vi "InitObjects.vi"(0 "Stand":refnum<class "Stand.lvclass">, 11 "error in":errorcluster, 13 "FPGA API":refnum<class "FPGA API.lvclass">) -> (4 "Stand out":refnum<class "Stand.lvclass">, 15 "error out":errorcluster)   [LabVIEW 2019, in "Stand.lvclass"]
uses:
  Stand.lvclass
  C:/Users/H4001/Documents/GitHub/H4000/src/Proccess_class/Proccess.lvclass
  C:/Users/H4001/Documents/GitHub/H4000/src/Device_class/Device.lvclass
  FPGA_API_class/FPGA API.lvclass
  Device_class/Device.lvclass/Device.ctl
  Proccess_class/Proccess.lvclass/Proccess.ctl
  AI_class/AI.lvclass
  Stand.lvclass/Stand.ctl
  Sig_DI_Simple_class/Sig_DI_Simple.lvclass
  MessageAMC_class/MessageAMC.lvclass
  C:/Users/H4001/Documents/GitHub/H4000/src/MessageInterface_class/MessageInterface.lvclass
  PM_Group_class/PM_Group.lvclass
  FPGA/TypeDef/DO index.ctl
  FPGA/TypeDef/DI index.ctl
  Valve_2DO_2DI_class/Valve_2DO_2DI.lvclass
  Proccess_class/Proccess.lvclass
  NeedleValve_class/NeedleValve.lvclass
  Device_class/Device.lvclass
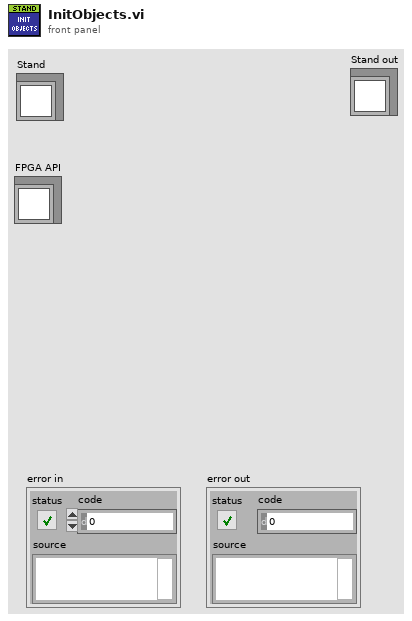
[diagram p1: front panel]
types:
  T1 = enum16{"AI", "DI", "NV", "PM", "VLV 44.1 44.2"}[]
  T2 = typedef "DI index.ctl" = u8
  T3 = typedef "DO index.ctl" = u8
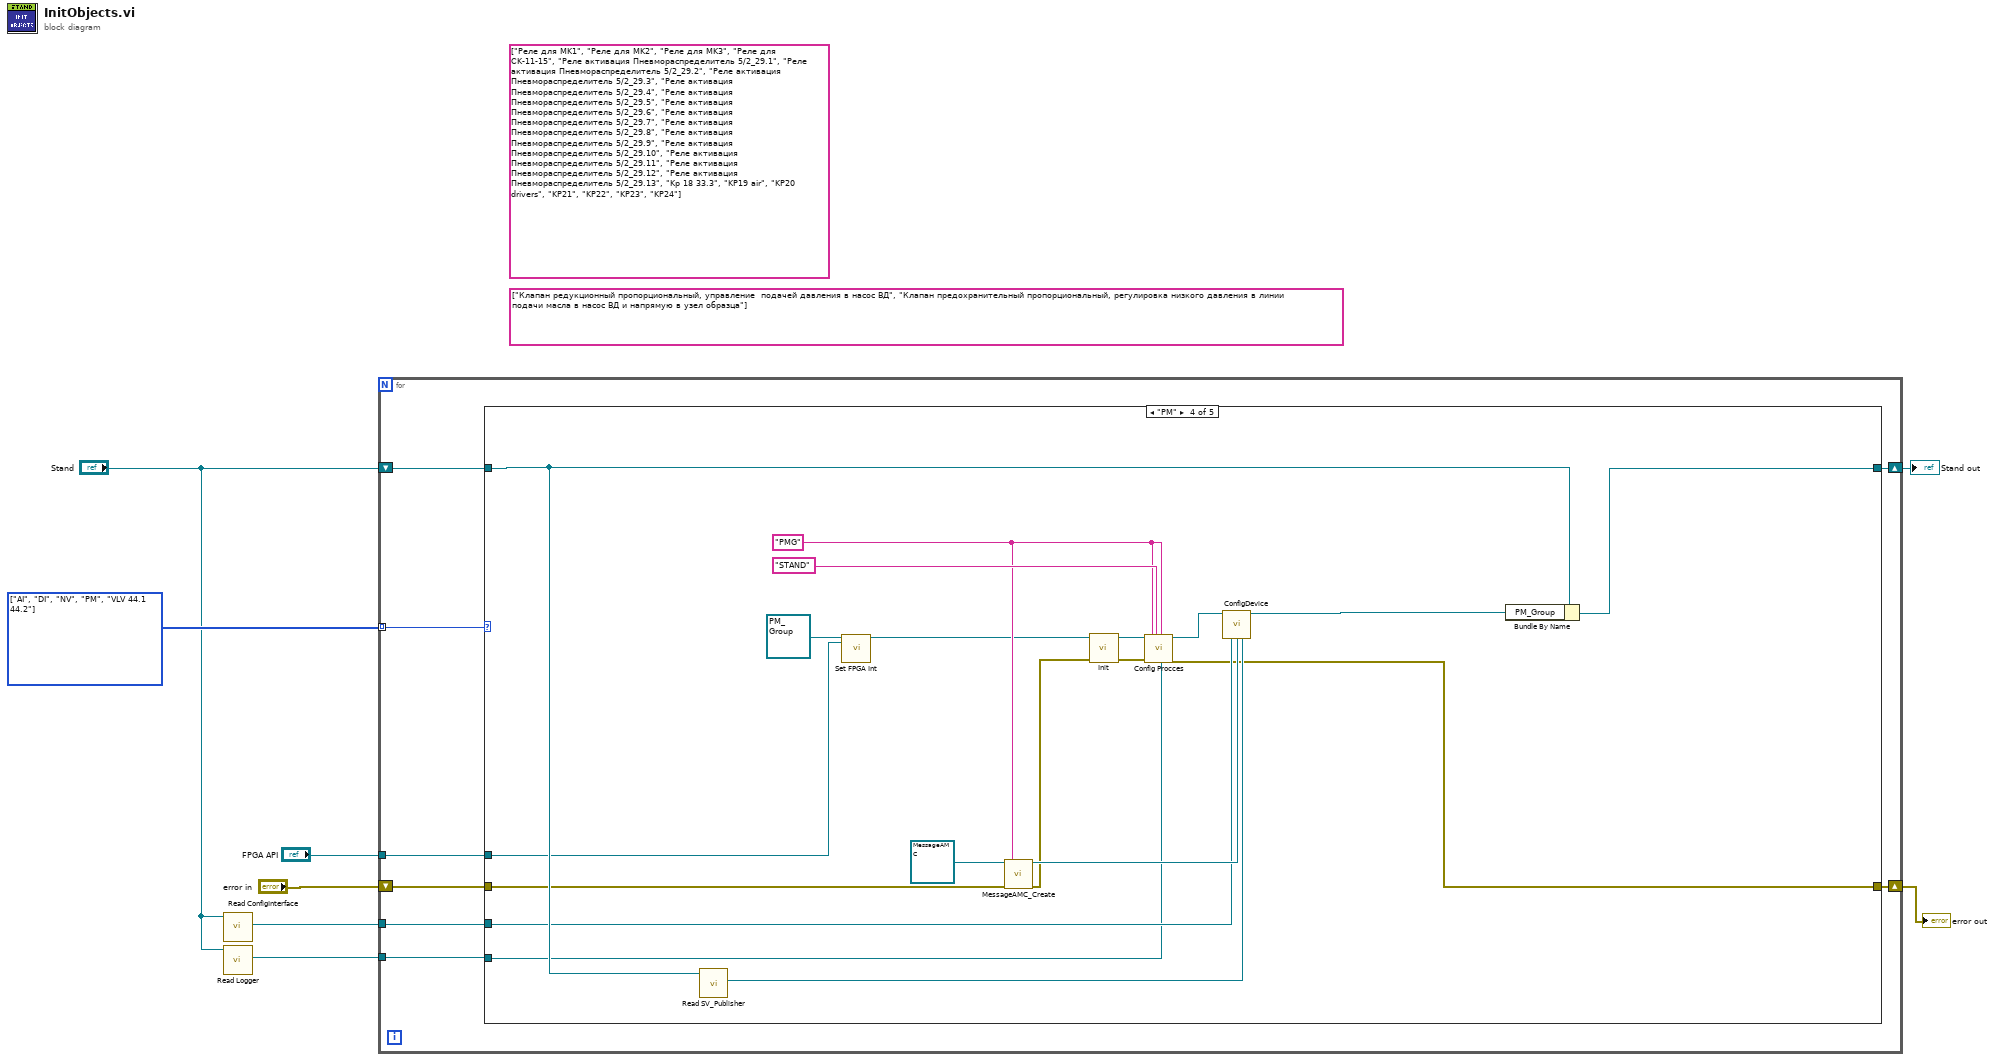
[diagram p0: block diagram]
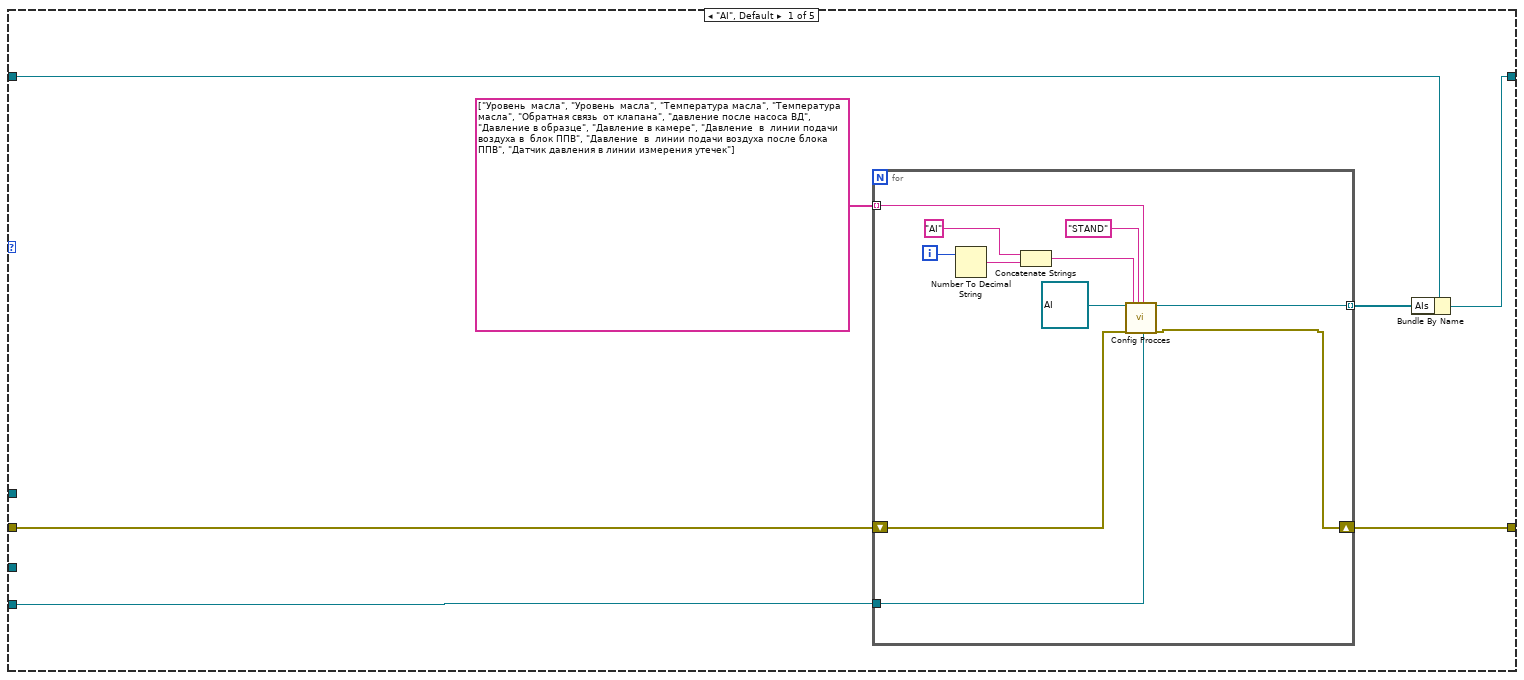
[diagram p2: hidden frame]
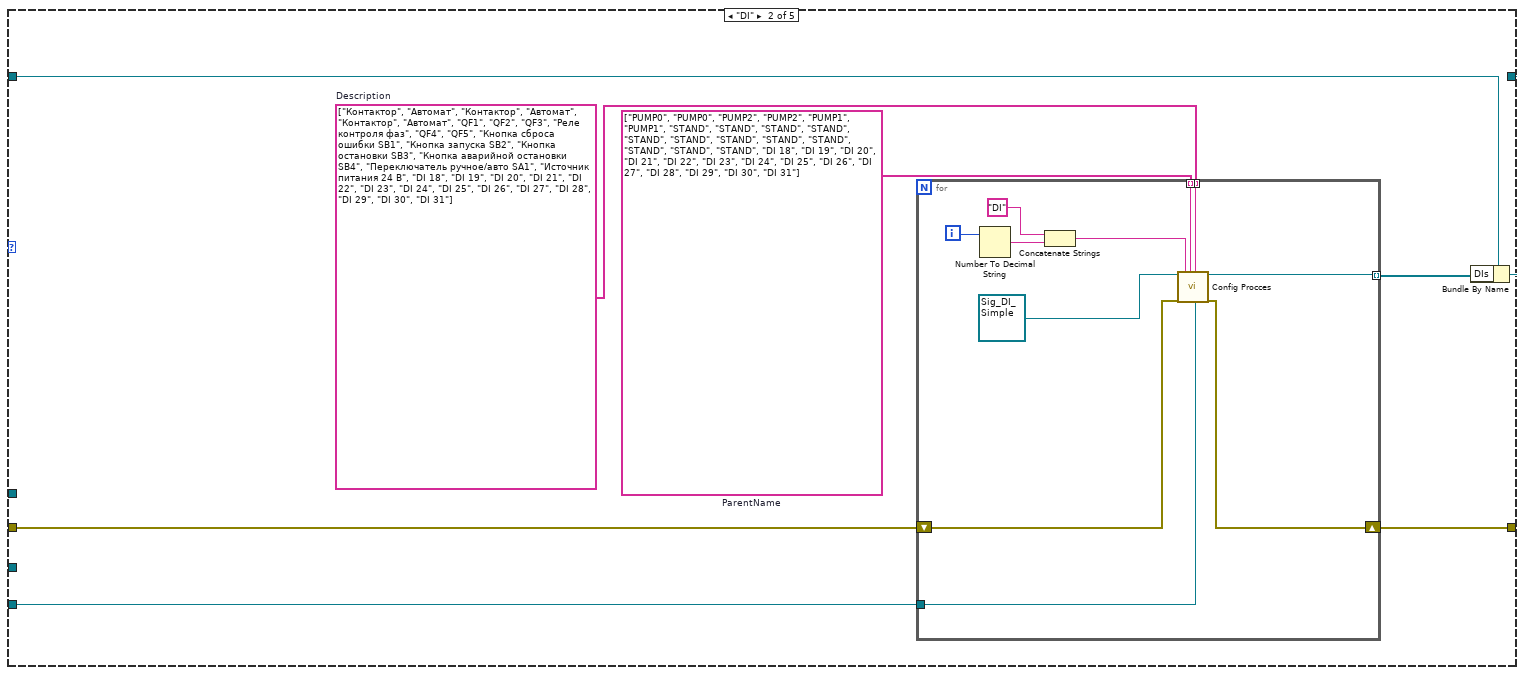
[diagram p3: hidden frame]
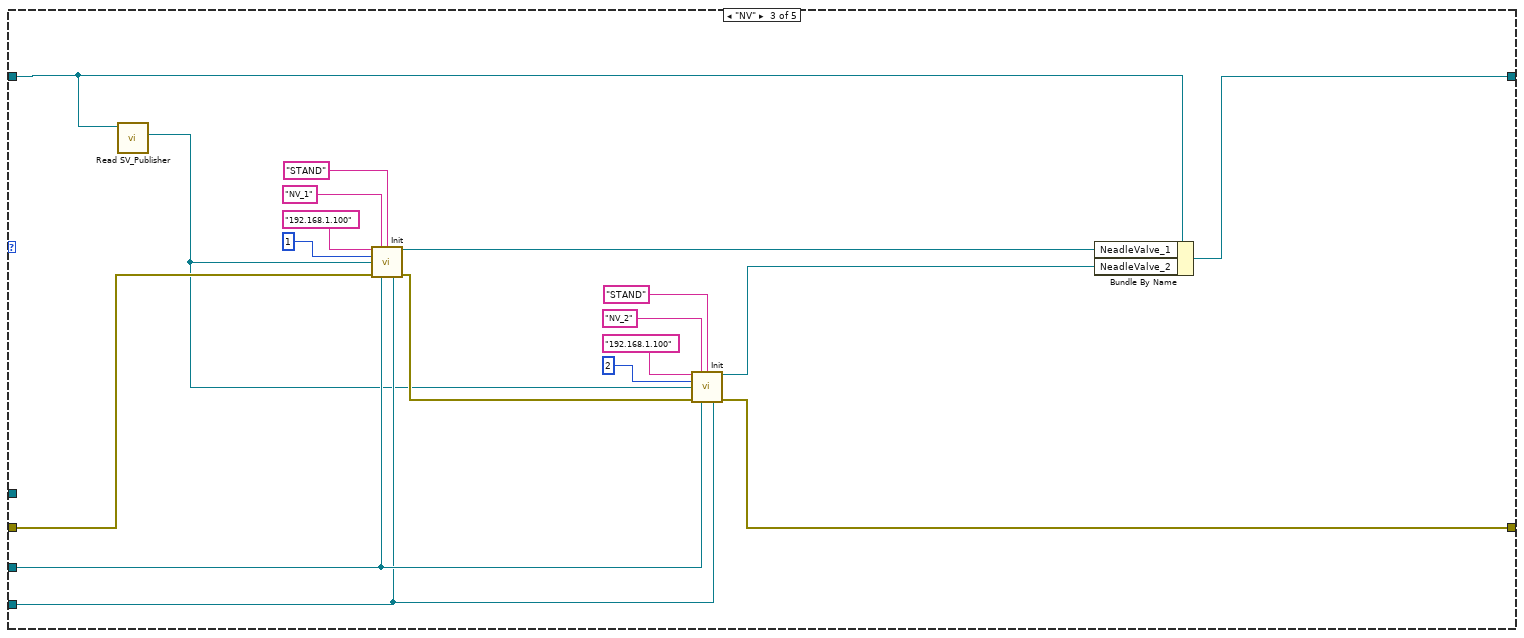
[diagram p4: hidden frame]
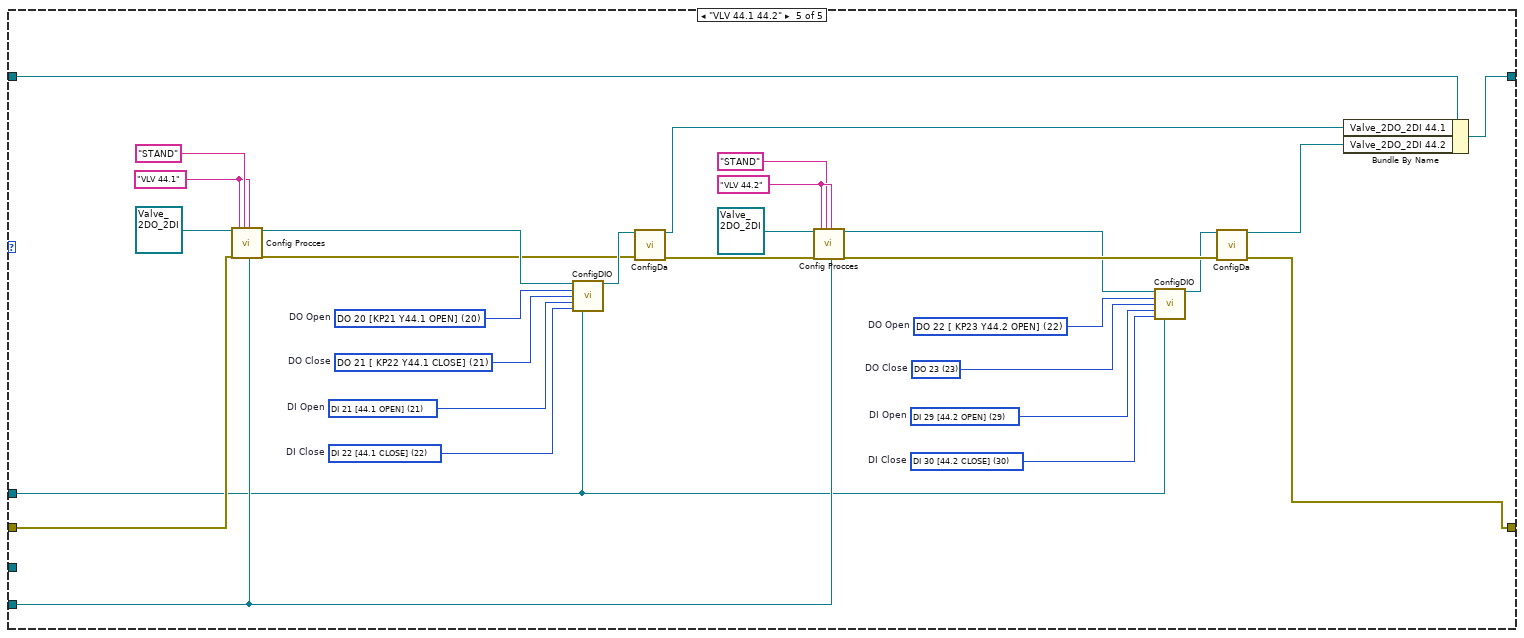
[diagram p5: hidden frame]
diagram:
  (unwired) string[] ["Реле для MK1", "Реле для MK2", "Реле для MK3", "Реле для CK-11-15", "Реле активация Пневмораспределитель 5/2_29.1", "Реле активация Пневмораспределитель 5/2_29.2", "Реле активация Пневмораспределитель 5/2_29.3", "Реле активация Пневмораспределитель 5/2_29.4", "Реле активация Пневмораспределитель 5/2_29.5", "Реле активация Пневмораспределитель 5/2_29.6", "Реле активация Пневмораспределитель 5/2_29.7", "Реле активация Пневмораспределитель 5/2_29.8", "Реле активация Пневмораспределитель 5/2_29.9", "Реле активация Пневмораспределитель 5/2_29.10", "Реле активация Пневмораспределитель 5/2_29.11", "Реле активация Пневмораспределитель 5/2_29.12", "Реле активация Пневмораспределитель 5/2_29.13", "Kp 18 33.3", "KP19 air", "KP20 drivers", "KP21", "KP22", "KP23", "KP24"] ("string array")
  (unwired) string[] ["Клапан редукционный пропорциональный, управление  подачей давления в насос ВД", "Клапан предохранительный пропорциональный, регулировка низкого давления в линии подачи масла в насос ВД и напрямую в узел образца"] ("ParentName")
  w8 = T1 [enum."AI", enum."DI", enum."NV", enum."PM", enum."VLV 44.1 44.2"] items=["AI", "DI", "NV", "PM", "VLV 44.1 44.2"]
  n1 = call "Read ConfigInterface.vi"("Device in"="Stand") -> ("ConfigInterface"=w2:refnum<class "ConfigInterface.lvclass">)  [unwired: 10 in]
  n2 = call "Read Logger.vi"("Proccess in"="Stand") -> ("Logger"=w4:refnum<class "Logger.lvclass">)  [unwired: 10 in]
  n3 = for {
    tunnel: w4 -> [w16]
    tunnel: w8 -> [w15] mode=indexing
    shift-right: [w14] -> w6
    shift-left: "error in" -> [w13]
    shift-right: [w11] -> w5
    shift-left: "Stand" -> [w12]
    tunnel: w2 -> [w10]
    tunnel: "FPGA API" -> [w9]
    n4 = case shown="\"PM\"" w15 {
      tunnel: [w23 w38 w56 w78 w96] -> w14
      tunnel: w16 -> [w22 w37 w58 w77 w92]
      tunnel: w13 -> [w21 w41 w65 w83 w109]
      tunnel: w12 -> [w20 w42 w55 w89 w119]
      tunnel: [w19 w40 w71 w90 w95] -> w11
      tunnel: w10 -> [_ _ w59 w81 _]
      tunnel: w9 -> [_ _ _ w72 w91]
      frame "AI", Default {
        n5 = for {
          tunnel: [w25] -> w18 mode=indexing
          shift-right: [w24] -> w23
          shift-left: w21 -> [w32]
          tunnel: w22 -> [w29]
          tunnel: string[] ["Уровень  масла", "Уровень  масла", "Температура масла", "Температура масла", "Обратная связь  от клапана", "давление после насоса ВД", "Давление в образце", "Давление в камере", "Давление  в  линии подачи воздуха в  блок ППВ", "Давление  в  линии подачи воздуха после блока ППВ", "Датчик давления в линии измерения утечек"] ("ParentName") -> [w27] mode=indexing
          i -> [w34]
          n6 = Number To Decimal String(number=w34) -> (decimal integer string=w33:string)  [unwired: 1 in]
          n7 = Concatenate Strings("AI" ("string"), w33) -> (w28:string)
          n8 = call "Config Procces.vi"("reference in"=refnum<class "AI.lvclass"> refnum ("Sig_AI"), "error in (no error)"=w32, "Name"=w28, "ParentName"="STAND", "Description"=w27, "Logger"=w29) -> ("reference out"=w25:refnum<class "AI.lvclass">, "error out"=w24:errorcluster)  [unwired: 12 in]
        }
        n9 = Bundle By Name(cluster=w20, "AIs"=w18) -> (w19:refnum<class "Stand.lvclass">)
      }
      frame "DI" {
        w35 = string[] ["PUMP0", "PUMP0", "PUMP2", "PUMP2", "PUMP1", "PUMP1", "STAND", "STAND", "STAND", "STAND", "STAND", "STAND", "STAND", "STAND", "STAND", "STAND", "STAND", "STAND", "DI 18", "DI 19", "DI 20", "DI 21", "DI 22", "DI 23", "DI 24", "DI 25", "DI 26", "DI 27", "DI 28", "DI 29", "DI 30", "DI 31"]  # ParentName
        w36 = string[] ["Контактор", "Автомат", "Контактор", "Автомат", "Контактор", "Автомат", "QF1", "QF2", "QF3", "Реле контроля фаз", "QF4", "QF5", "Кнопка сброса ошибки SB1", "Кнопка запуска SB2", "Кнопка остановки SB3", "Кнопка аварийной остановки SB4", "Переключатель ручное/авто SA1", "Источник питания 24 В", "DI 18", "DI 19", "DI 20", "DI 21", "DI 22", "DI 23", "DI 24", "DI 25", "DI 26", "DI 27", "DI 28", "DI 29", "DI 30", "DI 31"]  # Description
        n10 = for {
          tunnel: [w49] -> w39 mode=indexing
          shift-right: [w48] -> w38
          shift-left: w41 -> [w50]
          tunnel: w37 -> [w47]
          tunnel: w36 -> [w45] mode=indexing
          tunnel: w35 -> [w44] mode=indexing
          i -> [w53]
          n11 = Number To Decimal String(number=w53) -> (decimal integer string=w52:string)  [unwired: 1 in]
          n12 = Concatenate Strings("DI" ("string"), w52) -> (w46:string)
          n13 = call "Config Procces.vi"("reference in"=refnum<class "Sig_DI_Simple.lvclass"> refnum ("Sig_DI"), "error in (no error)"=w50, "Name"=w46, "ParentName"=w44, "Description"=w45, "Logger"=w47) -> ("reference out"=w49:refnum<class "Sig_DI_Simple.lvclass">, "error out"=w48:errorcluster)  [unwired: 12 in]
        }
        n14 = Bundle By Name(cluster=w42, "DIs"=w39) -> (w40:refnum<class "Stand.lvclass">)
      }
      frame "NV" {
        n15 = call "Read SV_Publisher.vi"("Device in"=w55) -> ("SV_Publisher.lvclass"=w54:refnum<class "SV_Publisher.lvclass">)  [unwired: 10 in]
        n16 = call "Init.vi"("address"="192.168.1.100", "Name"="NV_1", "ParentName"="STAND", "addres"=u16 1, "SV_Publisher"=w54, "error in (no error)"=w65, "ConfigInterface"=w59, "Logger"=w58) -> ("NeedleValve out"=w66:refnum<class "NeedleValve.lvclass">, "error out"=w60:errorcluster)  [unwired: 6 in]
        n17 = call "Init.vi"("address"="192.168.1.100", "Name"="NV_2", "ParentName"="STAND", "addres"=u16 2, "SV_Publisher"=w54, "error in (no error)"=w60, "ConfigInterface"=w59, "Logger"=w58) -> ("NeedleValve out"=w57:refnum<class "NeedleValve.lvclass">, "error out"=w56:errorcluster)  [unwired: 6 in]
        n18 = Bundle By Name(cluster=w55, "NeadleValve_1"=w66, "NeadleValve_2"=w57) -> (w71:refnum<class "Stand.lvclass">)
      }
      frame "PM" {
        w86 = "PMG" ("Name")
        n19 = call "Read SV_Publisher.vi"("Device in"=w89) -> ("SV_Publisher.lvclass"=w82:refnum<class "SV_Publisher.lvclass">)  [unwired: 10 in]
        n20 = call "Set FPGA Int.vi"("reference in"=refnum<class "PM_Group.lvclass"> refnum ("PM_Group in"), "FPGA API"=w72) -> ("reference out"=w73:refnum<class "PM_Group.lvclass">)  [unwired: 17 in]
        n21 = call "MessageAMC_Create.vi"("reference in"=refnum<class "MessageAMC.lvclass"> refnum, "error in (no error)"=w83, "message queue name"=w86) -> ("amc"=w84:refnum<class "MessageAMC.lvclass">, "error out"=w76:errorcluster)  [unwired: 15 in]
        n22 = call "Init.vi"("error in (no error)"=w76, "PM_Group in"=w73) -> ("error out"=w75:errorcluster, "PM_Group out"=w80:refnum<class "PM_Group.lvclass">)  [unwired: 8 in]
        n23 = call "Config Procces.vi"("reference in"=w80, "error in (no error)"=w75, "Name"=w86, "ParentName"="STAND", "Description"=w86, "Logger"=w77) -> ("reference out"=w85:refnum<class "PM_Group.lvclass">, "error out"=w78:errorcluster)  [unwired: 12 in]
        n24 = call "ConfigDevice.vi"("Device in"=w85, "ConfigInterface"=w81, "MessageInterface"=w84, "SV_Publisher"=w82) -> ("Device out"=w79:refnum<class "PM_Group.lvclass">)  [unwired: 11 in]
        n25 = Bundle By Name(cluster=w89, "PM_Group"=w79) -> (w90:refnum<class "Stand.lvclass">)
      }
      frame "VLV 44.1 44.2" {
        w106 = T2 30 items=["DI 0 [QF1]", "DI 1 [QF2]", "DI 2 [QF3]", "DI 3 [QF4]", "DI 4 [QF5]", "DI 5 [QF6]", "DI 6 [QF7]", "DI 7 [QF8]", "DI 8 [QF9]", "DI 9 [PHASE CONTROL RELAY CONTACTOR [KV1]]", "DI 10 [G1]", "DI 11 [G2]", "DI 12 [RESET BTN [SB1]]", "DI 13 [START BTN [SB2]]", "DI 14 [STOP BTN [SB3]]", "DI 15 [ES BTN [SB4]]", "DI 16 [MANUAL/AUTO MODE SA1]", "DI 17 [[S1]]", "DI 18 [[S2]]", "DI 19 [[S3]]", "DI 20 [[S4]]", "DI 21 [44.1 OPEN]", "DI 22 [44.1 CLOSE]", "DI 23 [CONTACTOR [MK1]] M12", "DI 24 [AUTOMATIC [QF11]] M12", "DI 25 [CONTACTOR [MK2]] M21", "DI 26 [AUTOMATIC [QF12]] M21", "DI 27 [CONTACTOR [MK3]] M24", "DI 28 [AUTOMATIC [QF13]] M24", "DI 29 [44.2 OPEN]", "DI 30 [44.2 CLOSE]"]  # DI Close
        w105 = T2 29 items=["DI 0 [QF1]", "DI 1 [QF2]", "DI 2 [QF3]", "DI 3 [QF4]", "DI 4 [QF5]", "DI 5 [QF6]", "DI 6 [QF7]", "DI 7 [QF8]", "DI 8 [QF9]", "DI 9 [PHASE CONTROL RELAY CONTACTOR [KV1]]", "DI 10 [G1]", "DI 11 [G2]", "DI 12 [RESET BTN [SB1]]", "DI 13 [START BTN [SB2]]", "DI 14 [STOP BTN [SB3]]", "DI 15 [ES BTN [SB4]]", "DI 16 [MANUAL/AUTO MODE SA1]", "DI 17 [[S1]]", "DI 18 [[S2]]", "DI 19 [[S3]]", "DI 20 [[S4]]", "DI 21 [44.1 OPEN]", "DI 22 [44.1 CLOSE]", "DI 23 [CONTACTOR [MK1]] M12", "DI 24 [AUTOMATIC [QF11]] M12", "DI 25 [CONTACTOR [MK2]] M21", "DI 26 [AUTOMATIC [QF12]] M21", "DI 27 [CONTACTOR [MK3]] M24", "DI 28 [AUTOMATIC [QF13]] M24", "DI 29 [44.2 OPEN]", "DI 30 [44.2 CLOSE]"]  # DI Open
        w104 = T3 23 items=["DO 0 [KP1] [M12]", "DO 1 [ON KP2] [M21]", "DO 2 [ON KP3] [M24]", "DO 3 [WATER Y18.1 [DO3]]", "DO 4 [WATER Y18.2 [DO4]]", "DO 5 [KP6 Y29.1 33.7]", "DO 6 [KP7 Y29.2 33.8]", "DO 7 [KP8 Y29.3 33.9]", "DO 8 [KP9 Y29.4  33.12]", "DO 9 [KP10 Y29.5 33.1]", "DO 10 [KP11 Y29.6 33.2]", "DO 11 [KP12 Y29.7  33.13]", "DO 12 [KP13 Y29.8  33.11]", "DO 13 [KP14 Y29.9 33.10]", "DO 14 [KP15 Y29.10  33.6]", "DO 15 [KP16 Y29.11  33.5]", "DO 16 [KP17 Y29.12  33.4]", "DO 17 [KP18 Y29.13 33.3]", "DO 18 [AIR KP19]", "DO 19 [STEP DRIVE EN KP20]", "DO 20 [KP21 Y44.1 OPEN]", "DO 21 [ KP22 Y44.1 CLOSE]", "DO 22 [ KP23 Y44.2 OPEN]", "DO 23", "DO 24 [STEP DRIVE 1]", "DO 25 [STEP DRIVE 2]"]  # DO Close
        w103 = T3 22 items=["DO 0 [KP1] [M12]", "DO 1 [ON KP2] [M21]", "DO 2 [ON KP3] [M24]", "DO 3 [WATER Y18.1 [DO3]]", "DO 4 [WATER Y18.2 [DO4]]", "DO 5 [KP6 Y29.1 33.7]", "DO 6 [KP7 Y29.2 33.8]", "DO 7 [KP8 Y29.3 33.9]", "DO 8 [KP9 Y29.4  33.12]", "DO 9 [KP10 Y29.5 33.1]", "DO 10 [KP11 Y29.6 33.2]", "DO 11 [KP12 Y29.7  33.13]", "DO 12 [KP13 Y29.8  33.11]", "DO 13 [KP14 Y29.9 33.10]", "DO 14 [KP15 Y29.10  33.6]", "DO 15 [KP16 Y29.11  33.5]", "DO 16 [KP17 Y29.12  33.4]", "DO 17 [KP18 Y29.13 33.3]", "DO 18 [AIR KP19]", "DO 19 [STEP DRIVE EN KP20]", "DO 20 [KP21 Y44.1 OPEN]", "DO 21 [ KP22 Y44.1 CLOSE]", "DO 22 [ KP23 Y44.2 OPEN]", "DO 23", "DO 24 [STEP DRIVE 1]", "DO 25 [STEP DRIVE 2]"]  # DO Open
        w100 = "VLV 44.2" ("string")
        w110 = T2 22 items=["DI 0 [QF1]", "DI 1 [QF2]", "DI 2 [QF3]", "DI 3 [QF4]", "DI 4 [QF5]", "DI 5 [QF6]", "DI 6 [QF7]", "DI 7 [QF8]", "DI 8 [QF9]", "DI 9 [PHASE CONTROL RELAY CONTACTOR [KV1]]", "DI 10 [G1]", "DI 11 [G2]", "DI 12 [RESET BTN [SB1]]", "DI 13 [START BTN [SB2]]", "DI 14 [STOP BTN [SB3]]", "DI 15 [ES BTN [SB4]]", "DI 16 [MANUAL/AUTO MODE SA1]", "DI 17 [[S1]]", "DI 18 [[S2]]", "DI 19 [[S3]]", "DI 20 [[S4]]", "DI 21 [44.1 OPEN]", "DI 22 [44.1 CLOSE]", "DI 23 [CONTACTOR [MK1]] M12", "DI 24 [AUTOMATIC [QF11]] M12", "DI 25 [CONTACTOR [MK2]] M21", "DI 26 [AUTOMATIC [QF12]] M21", "DI 27 [CONTACTOR [MK3]] M24", "DI 28 [AUTOMATIC [QF13]] M24", "DI 29 [44.2 OPEN]", "DI 30 [44.2 CLOSE]"]  # DI Close
        w111 = T2 21 items=["DI 0 [QF1]", "DI 1 [QF2]", "DI 2 [QF3]", "DI 3 [QF4]", "DI 4 [QF5]", "DI 5 [QF6]", "DI 6 [QF7]", "DI 7 [QF8]", "DI 8 [QF9]", "DI 9 [PHASE CONTROL RELAY CONTACTOR [KV1]]", "DI 10 [G1]", "DI 11 [G2]", "DI 12 [RESET BTN [SB1]]", "DI 13 [START BTN [SB2]]", "DI 14 [STOP BTN [SB3]]", "DI 15 [ES BTN [SB4]]", "DI 16 [MANUAL/AUTO MODE SA1]", "DI 17 [[S1]]", "DI 18 [[S2]]", "DI 19 [[S3]]", "DI 20 [[S4]]", "DI 21 [44.1 OPEN]", "DI 22 [44.1 CLOSE]", "DI 23 [CONTACTOR [MK1]] M12", "DI 24 [AUTOMATIC [QF11]] M12", "DI 25 [CONTACTOR [MK2]] M21", "DI 26 [AUTOMATIC [QF12]] M21", "DI 27 [CONTACTOR [MK3]] M24", "DI 28 [AUTOMATIC [QF13]] M24", "DI 29 [44.2 OPEN]", "DI 30 [44.2 CLOSE]"]  # DI Open
        w112 = T3 21 items=["DO 0 [KP1] [M12]", "DO 1 [ON KP2] [M21]", "DO 2 [ON KP3] [M24]", "DO 3 [WATER Y18.1 [DO3]]", "DO 4 [WATER Y18.2 [DO4]]", "DO 5 [KP6 Y29.1 33.7]", "DO 6 [KP7 Y29.2 33.8]", "DO 7 [KP8 Y29.3 33.9]", "DO 8 [KP9 Y29.4  33.12]", "DO 9 [KP10 Y29.5 33.1]", "DO 10 [KP11 Y29.6 33.2]", "DO 11 [KP12 Y29.7  33.13]", "DO 12 [KP13 Y29.8  33.11]", "DO 13 [KP14 Y29.9 33.10]", "DO 14 [KP15 Y29.10  33.6]", "DO 15 [KP16 Y29.11  33.5]", "DO 16 [KP17 Y29.12  33.4]", "DO 17 [KP18 Y29.13 33.3]", "DO 18 [AIR KP19]", "DO 19 [STEP DRIVE EN KP20]", "DO 20 [KP21 Y44.1 OPEN]", "DO 21 [ KP22 Y44.1 CLOSE]", "DO 22 [ KP23 Y44.2 OPEN]", "DO 23", "DO 24 [STEP DRIVE 1]", "DO 25 [STEP DRIVE 2]"]  # DO Close
        w113 = T3 20 items=["DO 0 [KP1] [M12]", "DO 1 [ON KP2] [M21]", "DO 2 [ON KP3] [M24]", "DO 3 [WATER Y18.1 [DO3]]", "DO 4 [WATER Y18.2 [DO4]]", "DO 5 [KP6 Y29.1 33.7]", "DO 6 [KP7 Y29.2 33.8]", "DO 7 [KP8 Y29.3 33.9]", "DO 8 [KP9 Y29.4  33.12]", "DO 9 [KP10 Y29.5 33.1]", "DO 10 [KP11 Y29.6 33.2]", "DO 11 [KP12 Y29.7  33.13]", "DO 12 [KP13 Y29.8  33.11]", "DO 13 [KP14 Y29.9 33.10]", "DO 14 [KP15 Y29.10  33.6]", "DO 15 [KP16 Y29.11  33.5]", "DO 16 [KP17 Y29.12  33.4]", "DO 17 [KP18 Y29.13 33.3]", "DO 18 [AIR KP19]", "DO 19 [STEP DRIVE EN KP20]", "DO 20 [KP21 Y44.1 OPEN]", "DO 21 [ KP22 Y44.1 CLOSE]", "DO 22 [ KP23 Y44.2 OPEN]", "DO 23", "DO 24 [STEP DRIVE 1]", "DO 25 [STEP DRIVE 2]"]  # DO Open
        w116 = "VLV 44.1" ("string")
        n26 = call "Config Procces.vi"("reference in"=refnum<class "Valve_2DO_2DI.lvclass"> refnum ("Pump_1AI_1DO_2DI in"), "error in (no error)"=w109, "Name"=w116, "ParentName"="STAND", "Description"=w116, "Logger"=w92) -> ("reference out"=w115:refnum<class "Valve_2DO_2DI.lvclass">, "error out"=w108:errorcluster)  [unwired: 12 in]
        n27 = call "ConfigDIO.vi"("Pump_1AI_1DO_2DI in"=w115, "DO Open"=w113, "DO Close"=w112, "DI Open"=w111, "DI Close"=w110, "FPGA API"=w91) -> ("Pump_1AI_1DO_2DI out"=w114:refnum<class "Valve_2DO_2DI.lvclass">)  [unwired: 9 in]
        n28 = call "ConfigDa.vi"("Pump_1AI_1DO_2DI in"=w114, "error in (no error)"=w108) -> ("Pump_1AI_1DO_2DI out"=w94:refnum<class "Valve_2DO_2DI.lvclass">, "error out"=w97:errorcluster)  [unwired: 12 in]
        n29 = call "Config Procces.vi"("reference in"=refnum<class "Valve_2DO_2DI.lvclass"> refnum ("Pump_1AI_1DO_2DI in"), "error in (no error)"=w97, "Name"=w100, "ParentName"="STAND", "Description"=w100, "Logger"=w92) -> ("reference out"=w101:refnum<class "Valve_2DO_2DI.lvclass">, "error out"=w107:errorcluster)  [unwired: 12 in]
        n30 = call "ConfigDIO.vi"("Pump_1AI_1DO_2DI in"=w101, "DO Open"=w103, "DO Close"=w104, "DI Open"=w105, "DI Close"=w106, "FPGA API"=w91) -> ("Pump_1AI_1DO_2DI out"=w102:refnum<class "Valve_2DO_2DI.lvclass">)  [unwired: 9 in]
        n31 = call "ConfigDa.vi"("Pump_1AI_1DO_2DI in"=w102, "error in (no error)"=w107) -> ("Pump_1AI_1DO_2DI out"=w93:refnum<class "Valve_2DO_2DI.lvclass">, "error out"=w96:errorcluster)  [unwired: 12 in]
        n32 = Bundle By Name(cluster=w119, "Valve_2DO_2DI 44.1"=w94, "Valve_2DO_2DI 44.2"=w93) -> (w95:refnum<class "Stand.lvclass">)
      }
    }
  }
  "error out" <- w6
  "Stand out" <- w5
